vi "Initialize.vi"(0 "VISA resource name":refnum<visa-resource-name>, 1 "Serial Configuration":T1={"Baud Rate"=9600, "Parity"=2, "Data Bits"=8, "Flow Control"=0} {"Flow Control" items=["None", "XON/XOFF", "RTS/CTS", "XON/XOFF & RTS/CTS"]; "Data Bits" items=["7"=7, "8"=8]; "Parity" items=["None", "Odd", "Even"]; "Baud Rate" items=["1200"=1200, "2400"=2400, "4800"=4800, "9600"=9600, "19200"=19200, "38400"=38400]}, 2 "Enable Advanced Security (False)":bool, 3 "Function Name (0 : Setting)":i32(ring) items=["Setting", "Monitor"], 5 "ID Query (True)":bool=TRUE, 9 "User ID (\"\")":string, 11 "error in (no error)":errorcluster, 12 "User Name (\"admin\")":string="admin", 13 "Password (\"\")":string) -> (4 "VISA resource name out":refnum<visa-resource-name>, 15 "error out":errorcluster)   [LabVIEW 2011, in "Yokogawa DX Series.lvlib"]
doc: "Establishes communication with the instrument and optionally performs an instrument identification query. It also places the instrument in a default state needed for other instrument driver operations. Therefore, call this VI before calling other instrument driver VIs for this instrument. Generally, you need to call the <B>Initialize VI</B> only once at the beginning of an application."
uses:
  <instrlib>/Yokogawa DX Series/Yokogawa DX Series.lvlib
panel:
  # "(c) 2010 Yokogawa Electric Corporation.  ALL RIGHTS RESERVED."
  # "Except for TCP/IP or Serial is not supported."
  # "ID query is not supported for DX100/DX200 series. Because the instrument can not check ID."
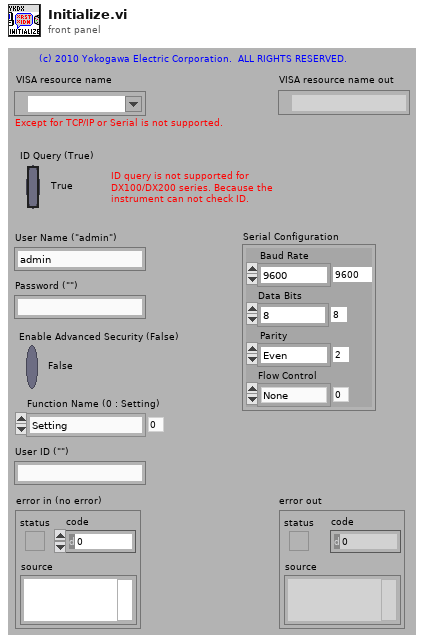
[diagram p1: front panel]
types:
  T1 = cluster{"Baud Rate":u32, "Parity":u16, "Data Bits":u16, "Flow Control":u16}
  T2 = cluster{"User Name":string, "User ID":string, "Password":string, "Model":i32}
  T3 = cluster{"Status":bool, "Code":i32, "Source (VI Name)":string}
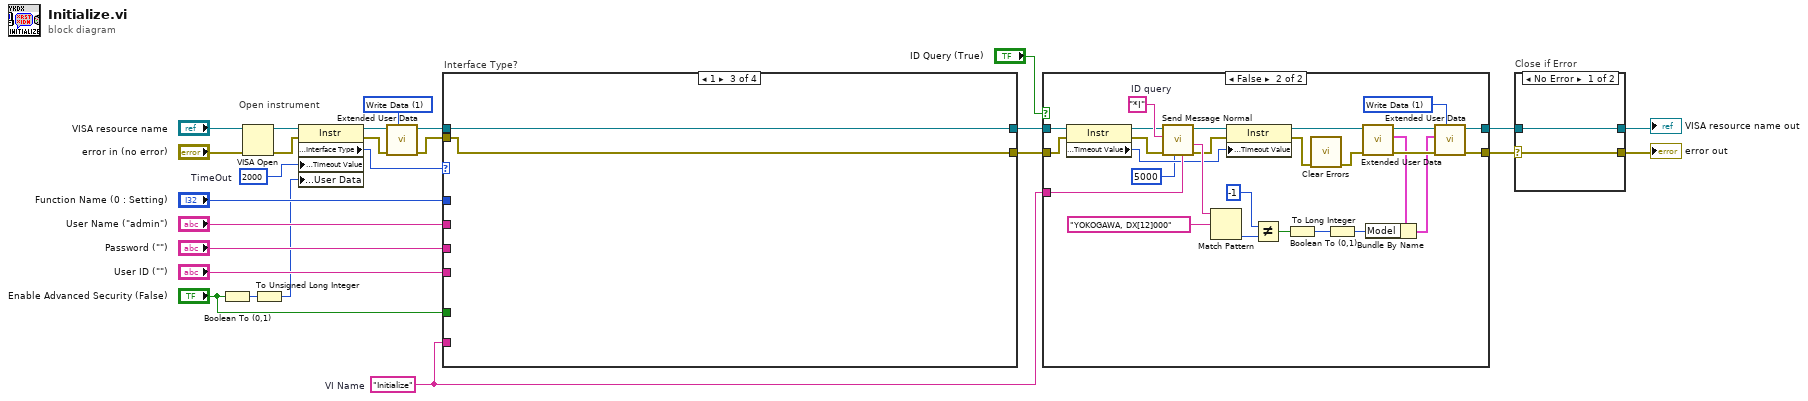
[diagram p0: block diagram]
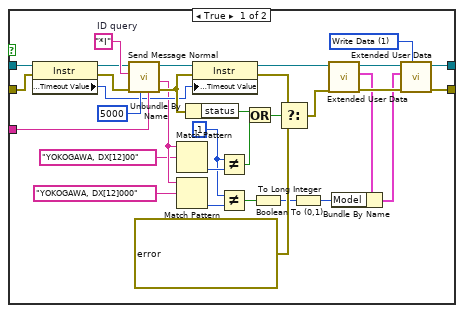
[diagram p2: hidden frame]
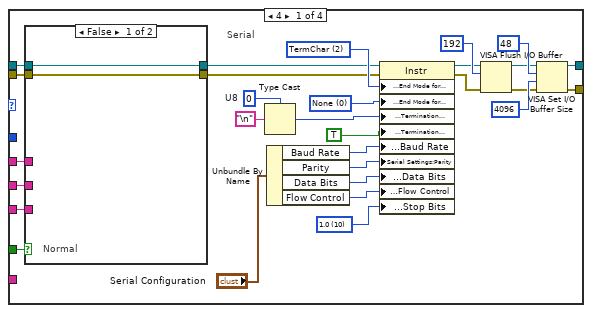
[diagram p3: hidden frame]
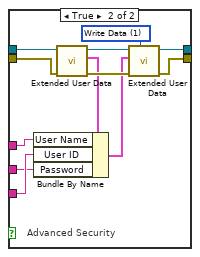
[diagram p4: hidden frame]
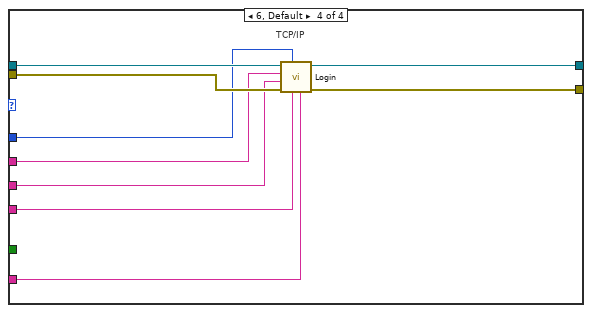
[diagram p6: hidden frame]
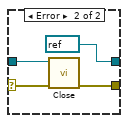
[diagram p7: hidden frame]
diagram:
  w2 = 1 items=["Read Data", "Write Data", "Clear Data", "Clear All Data"] ("Action")
  w1 = "Initialize"  # VI Name
  w19 = u32 2000  # TimeOut
  # "Open instrument"
  n1 = Boolean To (0,1)(Boolean="Enable Advanced Security (False)") -> (0, 1=w14:i16)
  n2 = VISA Open(error in (no error)="error in (no error)", VISA resource name="VISA resource name") -> (VISA resource name=w17:refnum<visa-resource-name>, error out=w24:errorcluster)  [unwired: 2 in, 1 out]
  n3 = To Unsigned Long Integer(number=w14) -> (unsigned 32bit integer=w13:u32)
  n4 = property class="Instr"(reference=w17, error in=w24, "General Settings:Timeout Value"=w19, "General Settings:User Data"=w13) -> (reference out=w6:refnum<visa-resource-name>, error out=w4:errorcluster, "Interface Information:Interface Type"=w18:u16)
  n5 = call <instrlib>:"Extended User Data.vi"("Action (0 : Read Data)"=w2, "error in (no error)"=w4, "VISA resource name"=w6) -> ("error out"=w3:errorcluster, "VISA resource name out"=w5:refnum<visa-resource-name>)  [unwired: 1 in, 6 out]
  n6 = case "Interface Type?" shown="1" w18 {
    tunnel: w5 -> [w41 w71 w73 w76]
    tunnel: [w31 w71 w73 w82] -> w11
    tunnel: w3 -> [w40 w70 w72 w79]
    tunnel: [w29 w70 w72 w81] -> w10
    tunnel: "User Name (\"admin\")" -> [w42 _ _ w77]
    tunnel: "Password (\"\")" -> [w43 _ _ w78]
    tunnel: w1 -> [_ _ _ w80]
    tunnel: "Function Name (0 : Setting)" -> [_ _ _ w75]
    tunnel: "User ID (\"\")" -> [w44 _ _ w74]
    tunnel: "Enable Advanced Security (False)" -> [w45 _ _ _]
    frame 4 {
      w48 = u16 10 items=["1.0"=10, "1.5"=15, "2.0"=20] ("Serial Settings:Stop Bits")
      w50 = u16 0 items=["None", "Last Bit", "TermChar", "Break"] ("Serial Settings:End Mode for Writes")
      w51 = u16 2 items=["None", "Last Bit", "TermChar"] ("Serial Settings:End Mode for Reads")
      w54 = u8 0  # U8
      # "Serial"
      n7 = case shown="False" w45 {
        tunnel: w44 -> [_ w59]
        tunnel: w43 -> [_ w58]
        tunnel: w42 -> [_ w64]
        tunnel: w41 -> [w56 w63]
        tunnel: w40 -> [w57 w62]
        tunnel: [w56 w66] -> w39
        tunnel: [w57 w65] -> w38
        frame False {
          # "Normal"
        }
        frame True {
          w67 = 1 items=["Read Data", "Write Data", "Clear Data", "Clear All Data"] ("Action")
          # "Advanced Security"
          n8 = call <instrlib>:"Extended User Data.vi"("error in (no error)"=w62, "VISA resource name"=w63) -> ("error out"=w69:errorcluster, "User Data Out"=w60:T2, "VISA resource name out"=w61:refnum<visa-resource-name>)  [unwired: 2 in, 5 out]
          n9 = Bundle By Name(cluster=w60, "User Name"=w64, "User ID"=w59, "Password"=w58) -> (w68:T2)
          n10 = call <instrlib>:"Extended User Data.vi"("Action (0 : Read Data)"=w67, "error in (no error)"=w69, "User Data In"=w68, "VISA resource name"=w61) -> ("error out"=w65:errorcluster, "VISA resource name out"=w66:refnum<visa-resource-name>)  [unwired: 6 out]
        }
      }
      n11 = Type Cast(type=w54, x="\n") -> (*(type *) &x=w27:u8)
      n12 = Unbundle By Name("Serial Configuration") -> ("Baud Rate"=w52:u32, "Parity"=w49:u16, "Data Bits"=w46:u16, "Flow Control"=w28:u16)
      n13 = property class="Instr"(reference=w39, error in=w38, "Serial Settings:End Mode for Reads"=w51, "Serial Settings:End Mode for Writes"=w50, "Message Based Settings:Termination Character"=w27, "Message Based Settings:Termination Character Enable"=TRUE, "Serial Settings:Baud Rate"=w52, "Serial Settings:Parity"=w49, "Serial Settings:Data Bits"=w46, "Serial Settings:Flow Control"=w28, "Serial Settings:Stop Bits"=w48) -> (reference out=w32:refnum<visa-resource-name>, error out=w30:errorcluster)
      n14 = VISA Flush I/O Buffer(VISA resource name=w32, mask (16)=u16 192, error in (no error)=w30) -> (VISA resource name out=w33:refnum<visa-resource-name>, error out=w34:errorcluster)
      n15 = VISA Set I/O Buffer Size(VISA resource name=w33, mask (16)=u16 48, size (4096)=u32 4096 ("size (0)"), error in (no error)=w34) -> (VISA resource name out=w31:refnum<visa-resource-name>, error out=w29:errorcluster)
    }
    frame 5 {
    }
    frame 1 {
    }
    frame 6, Default {
      # "TCP/IP"
      n16 = call <instrlib>:"Login.vi"("Source (\"\")"=w80, "User ID (\"\")"=w74, "Function Name (0 : Setting)"=w75, "error in (no error)"=w79, "Password (\"\")"=w78, "User Name (\"admin\")"=w77, "VISA resource name"=w76) -> ("error out"=w81:errorcluster, "VISA resource name out"=w82:refnum<visa-resource-name>)  [unwired: 3 out]
    }
  }
  n17 = case shown="False" "ID Query (True)" {
    tunnel: [w105 w134] -> w7
    tunnel: [w107 w136] -> w8
    tunnel: w11 -> [w92 w121]
    tunnel: w10 -> [w90 w119]
    tunnel: w1 -> [w98 w126]
    frame True {
      w104 = 1 items=["Read Data", "Write Data", "Clear Data", "Clear All Data"] ("Action")
      w84 = -1
      w115 = "*I"  # ID query
      n18 = property class="Instr"(reference=w92, error in=w90) -> (reference out=w91:refnum<visa-resource-name>, error out=w89:errorcluster, "General Settings:Timeout Value"=w88:u32)
      n19 = call <instrlib>:"Send Message Normal.vi"("Source (\"\")"=w98, "Timeout (25000)"=u32 5000, "error in (no error)"=w89, "Send Message (\"\")"=w115, "VISA resource name"=w91) -> ("error out"=w95:errorcluster, "Read Buffer"=w87:string, "VISA resource name out"=w96:refnum<visa-resource-name>)  [unwired: 4 out]
      n20 = Match Pattern(string=w87, regular expression="YOKOGAWA, DX[12]00") -> (offset past match=w85:i32)  [unwired: 4 out]
      n21 = Match Pattern(string=w87, regular expression="YOKOGAWA, DX[12]000") -> (offset past match=w110:i32)  [unwired: 4 out]
      n22 = Unbundle By Name(w95) -> ("status"=w112:bool)
      n23 = property class="Instr"(reference=w96, error in=w95, "General Settings:Timeout Value"=w88) -> (reference out=w94:refnum<visa-resource-name>, error out=w93:errorcluster)
      n24 = Not Equal?(x=w84, y=w85) -> (x != y?=w83:bool)
      n25 = Not Equal?(x=w84, y=w110) -> (x != y?=w101:bool)
      n26 = Or(x=w112, y=w83) -> (x .or. y?=w113:bool)
      n27 = Boolean To (0,1)(Boolean=w101) -> (0, 1=w100:i16)
      n28 = Select(t=w93, s=w113, f=T3 {"Status"=TRUE, "Code"=-1074003951, "Source (VI Name)"="<ERR> YKDX Initialize\nThe ID Query failed.  This may mean that you selected the wrong instrument or your instrument did not respond.  You may also be using a model that is not officially supported by this driver.  If you are sure that you have selected the correct instrument and it is responding, try disabling the ID Query."}) -> (s? t:f=w109:T3)
      n29 = To Long Integer(number=w100) -> (32bit integer=w99:i32)
      n30 = call <instrlib>:"Extended User Data.vi"("error in (no error)"=w109, "VISA resource name"=w94) -> ("error out"=w106:errorcluster, "User Data Out"=w103:T2, "VISA resource name out"=w108:refnum<visa-resource-name>)  [unwired: 2 in, 5 out]
      n31 = Bundle By Name(cluster=w103, "Model"=w99) -> (w102:T2)
      n32 = call <instrlib>:"Extended User Data.vi"("Action (0 : Read Data)"=w104, "error in (no error)"=w106, "User Data In"=w102, "VISA resource name"=w108) -> ("error out"=w105:errorcluster, "VISA resource name out"=w107:refnum<visa-resource-name>)  [unwired: 6 out]
    }
    frame False {
      w133 = 1 items=["Read Data", "Write Data", "Clear Data", "Clear All Data"] ("Action")
      w142 = "*I"  # ID query
      n33 = property class="Instr"(reference=w121, error in=w119) -> (reference out=w120:refnum<visa-resource-name>, error out=w118:errorcluster, "General Settings:Timeout Value"=w117:u32)
      n34 = call <instrlib>:"Send Message Normal.vi"("Source (\"\")"=w126, "Timeout (25000)"=u32 5000, "error in (no error)"=w118, "Send Message (\"\")"=w142, "VISA resource name"=w120) -> ("error out"=w124:errorcluster, "Read Buffer"=w140:string, "VISA resource name out"=w125:refnum<visa-resource-name>)  [unwired: 4 out]
      n35 = Match Pattern(string=w140, regular expression="YOKOGAWA, DX[12]000") -> (offset past match=w138:i32)  [unwired: 4 out]
      n36 = property class="Instr"(reference=w125, error in=w124, "General Settings:Timeout Value"=w117) -> (reference out=w123:refnum<visa-resource-name>, error out=w122:errorcluster)
      n37 = Not Equal?(x=-1, y=w138) -> (x != y?=w130:bool)
      n38 = Boolean To (0,1)(Boolean=w130) -> (0, 1=w129:i16)
      n39 = call <vilib>:"Clear Errors.vi"("error in (no error)"=w122) -> ("error out"=w127:errorcluster)  [unwired: 6 out]
      n40 = To Long Integer(number=w129) -> (32bit integer=w128:i32)
      n41 = call <instrlib>:"Extended User Data.vi"("error in (no error)"=w127, "VISA resource name"=w123) -> ("error out"=w135:errorcluster, "User Data Out"=w132:T2, "VISA resource name out"=w137:refnum<visa-resource-name>)  [unwired: 2 in, 5 out]
      n42 = Bundle By Name(cluster=w132, "Model"=w128) -> (w131:T2)
      n43 = call <instrlib>:"Extended User Data.vi"("Action (0 : Read Data)"=w133, "error in (no error)"=w135, "User Data In"=w131, "VISA resource name"=w137) -> ("error out"=w134:errorcluster, "VISA resource name out"=w136:refnum<visa-resource-name>)  [unwired: 6 out]
    }
  }
  n44 = case "Close if Error" shown="No Error" w7 {
    selector: w7 -> [w143 w146]
    tunnel: w8 -> [w144 w147]
    tunnel: [w144 refnum<visa-resource-name> refnum ("VISA resource name out")] -> w26
    tunnel: [w143 w148] -> w25
    frame No Error {
    }
    frame Error {
      n45 = call <instrlib>:"Close.vi"("error in (no error)"=w146, "VISA resource name"=w147) -> ("error out"=w148:errorcluster)  [unwired: 9 out]
    }
  }
  "VISA resource name out" <- w26
  "error out" <- w25
